vi "Read Limit Switches.vi"(8 "error in (no error)":errorcluster, 11 "Hardware Settings in":refnum<class "Hardware Settings.lvclass">) -> (0 "error out":errorcluster, 2 "Limits":T1, 3 "Hardware Settings out":refnum<class "Hardware Settings.lvclass">)   [LabVIEW 2017, in "Expansion.lvclass"]
uses:
  Expansion.lvclass
  Hardware Settings/Hardware Settings.lvclass
  Type Defs/Limit Switches.ctl
  Hardware Settings/Type Defs/Hardware Types.ctl
  Hardware Settings/Hardware Types/Generic/Generic Hardware.lvclass
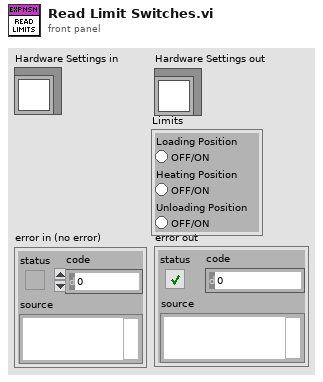
[diagram p1: front panel]
types:
  T1 = typedef "Expansion.lvclass/Limit Switches.ctl" = cluster{"Loading Position":bool, "Heating Position":bool, "Unloading Position":bool}
  T2 = typedef "Hardware Settings.lvclass/Hardware Types.ctl" = string
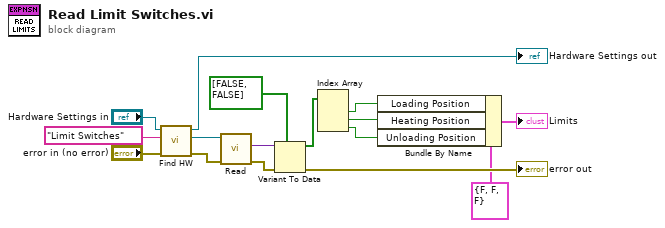
[diagram p0: block diagram]
diagram:
  n1 = call "Find HW.vi"("error in (no error)"="error in (no error)", "HW Item"=T2 "Limit Switches", "Hardware Settings in"="Hardware Settings in") -> ("error out"=w14:errorcluster, "Selected Hardware Out"=w11:refnum<class "Generic Hardware.lvclass">, "Hardware Settings out"=→"Hardware Settings out":refnum<class "Hardware Settings.lvclass">)  [unwired: 6 in]
  n2 = call-dynamic "Read.vi"("error in (no error)"=w14, "Generic Hardware in"=w11) -> ("error out"=w15:errorcluster, "Output"=w12:variant)  [unwired: 7 in, 1 out]
  n3 = Variant To Data(error in=w15, type=bool[] [FALSE, FALSE], Variant=w12) -> (data=w13:bool[], error out=→"error out":errorcluster)
  n4 = Index Array(array=w13) -> (element #1=w3:bool, element #2=w2:bool, element #3=w1:bool)  [unwired: 3 in]
  n5 = Bundle By Name(cluster=T1 {"Loading Position"=FALSE, "Heating Position"=FALSE, "Unloading Position"=FALSE} ("Limits 2"), "Loading Position"=w3, "Heating Position"=w2, "Unloading Position"=w1) -> (→"Limits":T1)
